vi "getTemperature.vi"(6 "Channel":i32, 8 "error in (no error)":errorcluster, 11 "instrument.Cryostation in":refnum<class "instrument.Cryostation.lvclass">) -> (0 "error out":errorcluster, 1 "Status":string, 2 "Temperature (K)":dbl, 3 "instrument.Cryostation out":refnum<class "instrument.Cryostation.lvclass">, 4 "Finished?":bool)   [LabVIEW 2019, in "instrument.Cryostation.lvclass"]
doc: "Returns the Montana Cryostation Temperature in (K)\n\n<b>Channels:</b>\n- 0: Sample\n- 1: Platform\n- 2: Stage 1\n- 3: Stage 2"
uses:
  instrument.Cryostation.lvclass
  <userlib>/LevyLab/Instrument Framework/Instrument Types/Cryostat/Instrument.Cryostat.lvclass
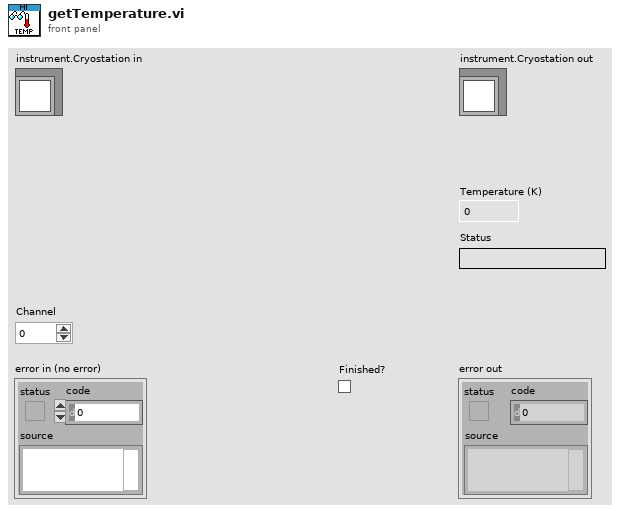
[diagram p1: front panel]
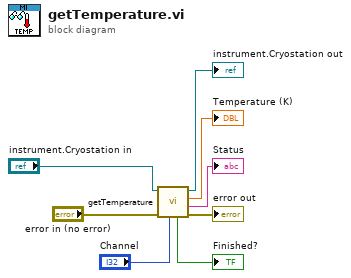
[diagram p0: block diagram]
diagram:
  n1 = call-parent "getTemperature.vi"("Channel"="Channel", "error in (no error)"="error in (no error)", "Instrument.Cryostat in"="instrument.Cryostation in") -> ("error out"=→"error out":errorcluster, "Status"=→"Status":string, "Temperature (K)"=→"Temperature (K)":dbl, "Instrument.Cryostat out"=→"instrument.Cryostation out":refnum<class "instrument.Cryostation.lvclass">, "Finished?"=→"Finished?":bool)  [unwired: 4 in]
